vi "hidSPD Write Report.vi"(8 "error in (no error)":errorcluster, 9 "data":i32[](array[numeric]), 10 "cmd":i32, 11 "spdDevSession in":T1 {"hidSPD.Sturtup Values"."HV_bias" format="%#_6p, V"; "hidSPD.Sturtup Values"."TSet" format="%#_6p, DegC"; "hidSPD.Controller"."HV_bias" format="%#_6p, V"; "hidSPD.Controller"."TSet" format="%#_6p, DegC"}) -> (0 "error out":errorcluster, 3 "spdDevSession out":T1 {"hidSPD.Sturtup Values"."HV_bias" format="%#_6p, V"; "hidSPD.Sturtup Values"."TSet" format="%#_6p, DegC"; "hidSPD.Controller"."HV_bias" format="%#_6p, V"; "hidSPD.Controller"."TSet" format="%#_6p, DegC"})   [LabVIEW 2018, in "hidSPDLibForLabView.lvlib"]
uses:
  hidSPDLibForLabView.lvlib
  hidSPD Controls/hidSPD Device Session.ctl
  hidSPD Controls/hidSPD Controller.ctl
  hidSPD Controls/hidSPD SPD Type.ctl
  <vilib>/Utility/error.llb/Error Cluster From Error Code.vi
  <vilib>/ErrorRing/Error Ring.xnode
  hidSPD DLL files/libSPD.dll
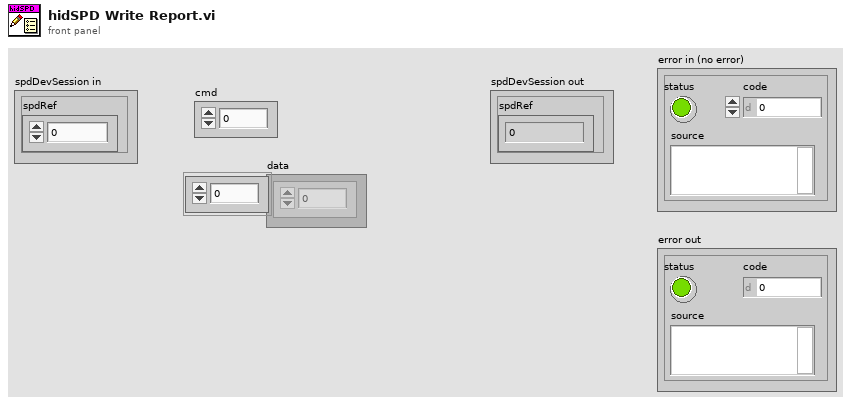
[diagram p1: front panel]
types:
  T1 = typedef "hidSPDLibForLabView.lvlib/hidSPD Device Session.ctl" = cluster{"spdRef":u64, "connected":bool, "spdName":string, "hidSPD.Controller":T2, "hidSPD.Sturtup Values":T2, "SPD Type":T3}
  T2 = typedef "hidSPDLibForLabView.lvlib/hidSPD Controller.ctl" = cluster{"TSet":sgl, "HV_bias":sgl, "DDS_stb_code":u16}
  T3 = typedef "hidSPDLibForLabView.lvlib/hidSPD SPD Type.ctl" = enum16{"Free Run", "Gate"}
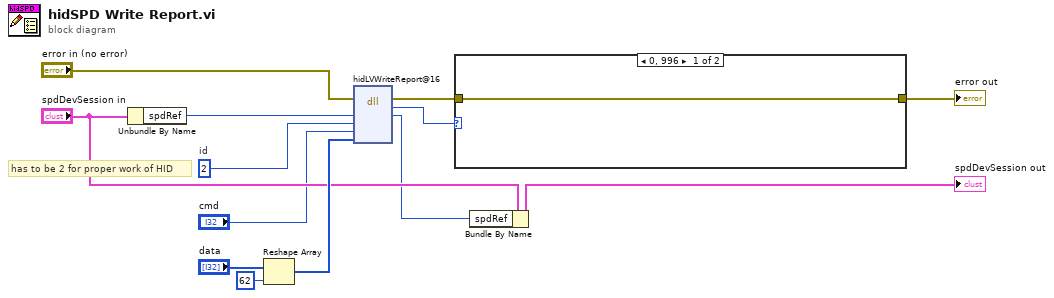
[diagram p0: block diagram]
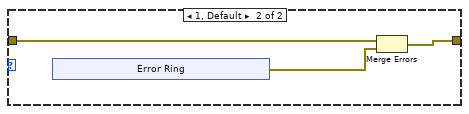
[diagram p2: hidden frame]
diagram:
  w7 = 2  # id
  # "has to be 2 for proper work of HID"
  n1 = Unbundle By Name("spdDevSession in") -> ("spdRef"=w3:u64)
  n2 = Reshape Array("data", 62 ("dimension size")) -> (w11:i32[])
  n3 = dll-call lib="D:/NextCloud/SPD stand/Automative SPD Measurements/Automative SPD Stand/Instruments/SPD HID Interface/hidSPDLibForLabView/hidSPD DLL files/libSPD.dll" fn="hidLVWriteReport@16"(error in="error in (no error)", "spdDeviceHandle"=w3, "id"=w7, "cmd"="cmd", "data"=w11) -> (error out=w5:errorcluster, "error"=w2:i32, "spdDeviceHandle"=w1:u64)  [unwired: 5 in, 1 out]
  n4 = case shown="0, 996" w2 {
    tunnel: [w14 w17] -> w4
    tunnel: w5 -> [w14 w16]
    frame 0, 996 {
    }
    frame 1, Default {
      n5 = xnode "Error Ring"() -> ("error out"=w15:errorcluster)
      n6 = Merge Errors(w16, w15) -> (w17:errorcluster)
    }
  }
  "error out" <- w4
  n7 = Bundle By Name(cluster="spdDevSession in", "spdRef"=w1) -> (→"spdDevSession out":T1)
